vi "Populate Worker Ring.vi"(8 "error in (no error)":errorcluster, 10 "Worker List":string[](array[string]), 11 "Task Setting Editor in":refnum<class "Task Setting Editor.lvclass">) -> (0 "error out":errorcluster, 3 "Task Setting Editor out":refnum<class "Task Setting Editor.lvclass">)   [LabVIEW 2017, in "Task Setting Editor.lvlib" / "Task Setting Editor.lvclass"]
uses:
  Task Setting Editor.lvclass
  Task Setting Editor.lvclass/Task Setting Editor.ctl
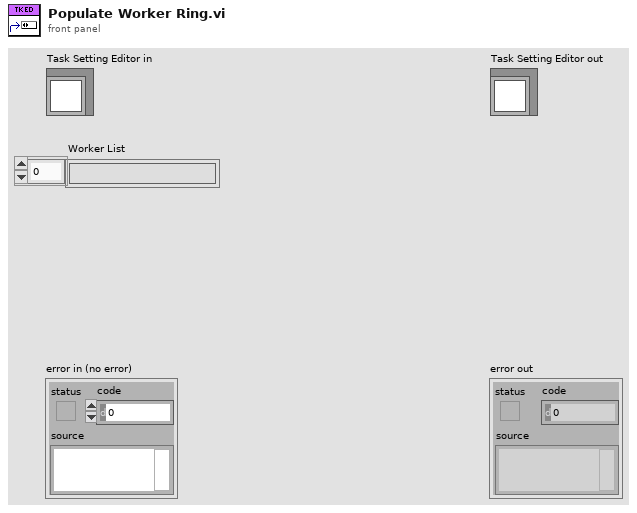
[diagram p1: front panel]
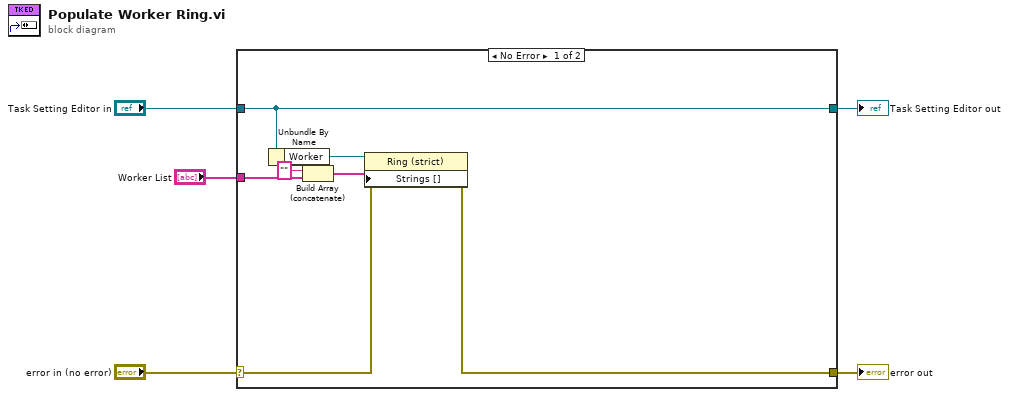
[diagram p0: block diagram]
diagram:
  n1 = case shown="No Error" "error in (no error)" {
    selector: "error in (no error)" -> [w9 w14]
    tunnel: [w8 w14] -> w4
    tunnel: [w12 w13] -> w2
    tunnel: "Task Setting Editor in" -> [w12 w13]
    tunnel: "Worker List" -> [w10 _]
    frame No Error {
      n2 = Unbundle By Name(w12) -> ("Worker"=w11:refnum<vi>)
      n3 = Build Array (concatenate)("", w10) -> (w7:string[])
      n4 = property class="Ring (strict)"(reference=w11, error in=w9, "Strings []"=w7) -> (error out=w8:errorcluster)  [unwired: 1 out]
    }
    frame Error {
    }
  }
  "error out" <- w4
  "Task Setting Editor out" <- w2
